vi "FPGA.vi"() -> ()   [LabVIEW 2017]
uses:
  <vilib>/Platform/TimedLoop/XDataNode/timing_clust.ctl
  <vilib>/Platform/TimedLoop/XDataNode/nitl_modes.ctl
  <vilib>/Platform/TimedLoop/XDataNode/wakeup.ctl
  <vilib>/rvi/Emulation/niFpgaGetClockAttributes.vi
  <vilib>/rvi/Emulation/niFpgaSctlEmulationGetInTimedLoop.vi
  <vilib>/rvi/Emulation/niFpgaEmulationReportErrorSimple.vi
  <vilib>/rvi/eio/common/nirviEmuTemplateMethod_errors.vi
  <vilib>/rvi/Emulation/niFpgaCriticalErrorInLSC.vi
  <vilib>/rvi/Emulation/niFpgaProcessEmulError.vi
  Control/GV FIFO timeout.vi
  Control/GV DO delay.vi
  Control/GV trigger delay.vi
  <vilib>/eio/EIONode/EIONode.xnode
  <vilib>/Platform/TimedLoop/XDataNode/XDataNode.xnode
  <vilib>/Platform/TimedLoop/XDataNode/XDNodeRunTimeDep.lvlib
  <vilib>/rvi/occurrence/nirviOccurrence.lvlib
  Detector/GV gated pixel clock change.vi
  Detector/GV line gate.vi
  Detector/GV pretrigger.vi
panel:
  in  "FIFO OUT debug":bool
  in  "PC1_voltage":i16
  in  "RS_voltage":i16
  in  "ON/OFF":bool
  in  "VT_NC":bool
  in  "VT_forward":bool
  in  "VT_back":bool
  in  "VT_start":bool
  in  "Sync_AODO_to_LineGate":u16
  in  "Start_acquisition":bool
  in  "Nmax_lines":u16=1
  in  "Pulse sequence":bool[](array[boolean])=[TRUE, FALSE, FALSE, FALSE, FALSE, FALSE, FALSE, FALSE, FALSE, FALSE, FALSE, FALSE, FALSE, FALSE, FALSE, FALSE, FALSE, FALSE, FALSE, FALSE]
  in  "Nchannels":u16=4
  in  "FIFO_timeout":u16=100
  in  "Trigger":bool
  in  "Sync_DO_to_AO":u16=296
  # "RESONANT\nSCANNER"
  # "POCKELS #1"
  # "VIBRATOME"
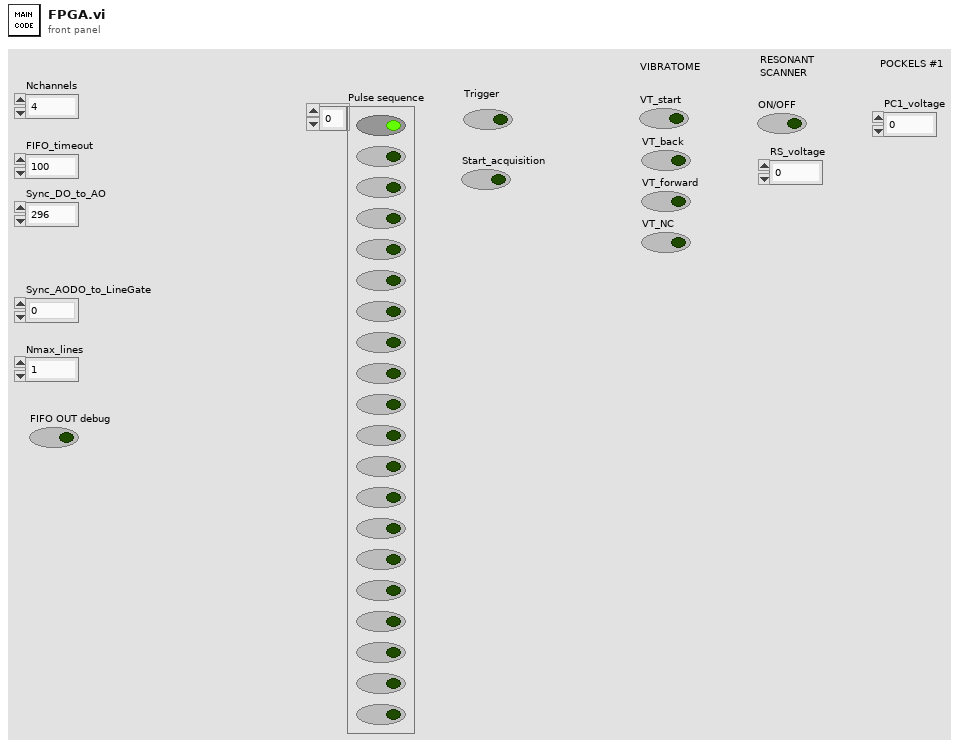
[diagram p1: front panel]
types:
  T1 = typedef "XDNodeRunTimeDep.lvlib/timing_clust.ctl" = cluster{"Expected End [f-1]":u64, "Actual End [f-1]":u64, "Finished Late? [f-1]":bool, "Expected End [i-1]":u64, "Actual End [i-1]":u64, "Finished Late? [i-1]":bool, "Expected Start [i]":u64, "Actual Start [i]":u64, "Expected Start [f]":u64, "Actual Start [f]":u64, "Source Name":string, "Structure Name":string, "Period":i64, "Deadline":i64, "Offset":i64, "Start":i64, "Priority":i32, "Timeout":i32, "Mode":T2, "Wakeup Reason":T3, "Error":errorcluster, "Source Type":string, "Secondary Source Type":string, "Global End Time":u64, "Global Start Time":u64, "Frame Duration":u64, "Iteration Duration":u64, "Assigned CPU":i32, "I/O Scan Engine Mode":u32}
  T2 = typedef "XDNodeRunTimeDep.lvlib/nitl_modes.ctl" = enum32{"No Change", "Process missed periods, maintain original phase", "Discard missed periods, maintain original phase", "Process missed periods, ignore original phase", "Discard missed periods, ignore original phase"}
  T3 = typedef "XDNodeRunTimeDep.lvlib/wakeup.ctl" = enum32{"Normal", "Aborted", "Asynchronous wakeup", "Timing source error", "Timed loop error", "Timeout"}
  T4 = cluster{"Pixel clock change":bool, "Line clock change":bool}
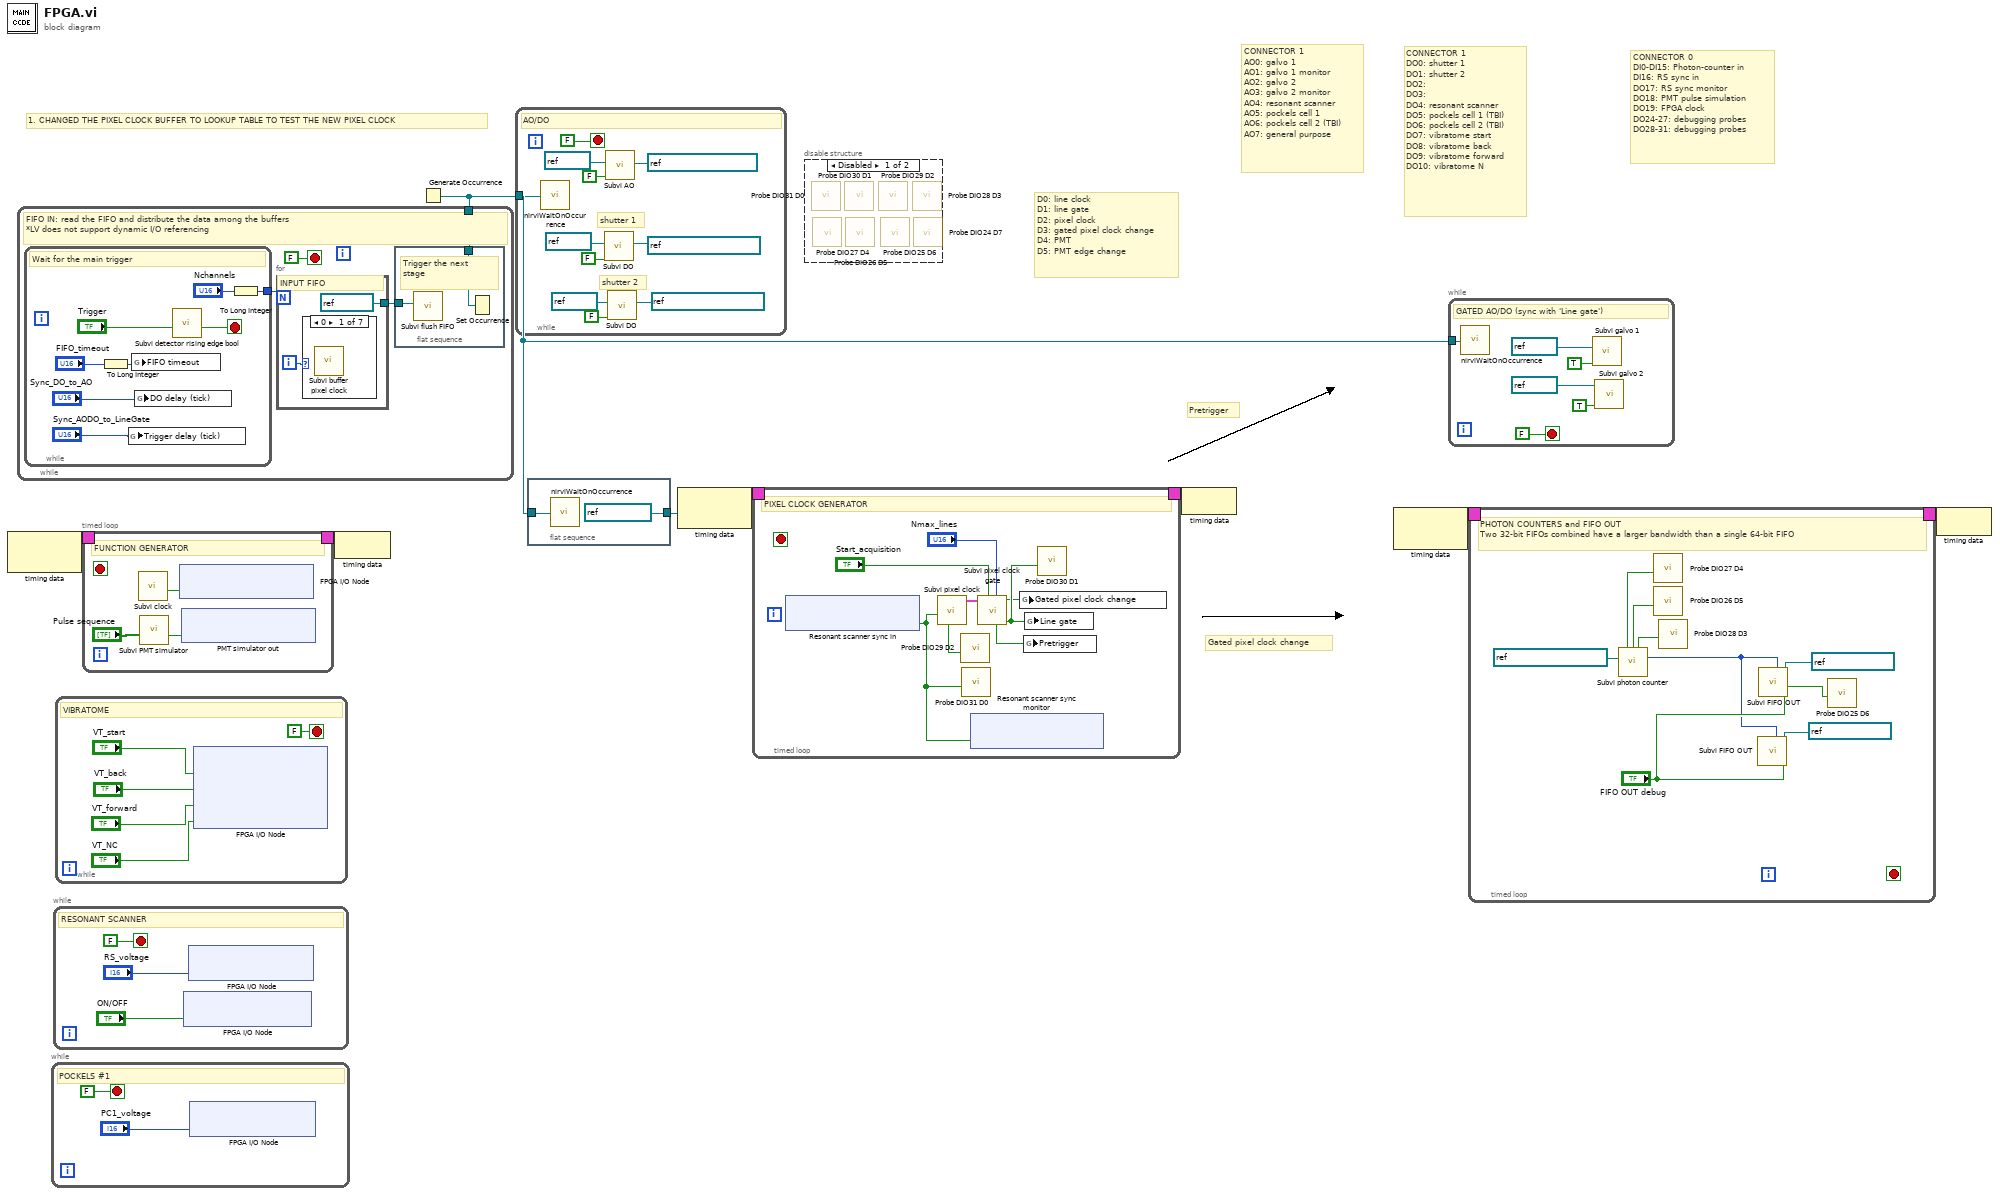
[diagram p0: block diagram]
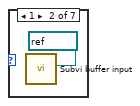
[diagram p3: hidden frame]
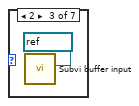
[diagram p4: hidden frame]
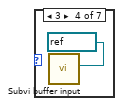
[diagram p5: hidden frame]
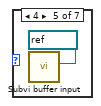
[diagram p6: hidden frame]
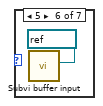
[diagram p7: hidden frame]
diagram:
  # "CONNECTOR 0\nDI0-DI15: Photon-counter in\nDI16: RS sync in \nDO17: RS sync monitor\nDO18: PMT pulse simulation\nDO19: FPGA clock\nDO24-27: debugging probes\nDO28-31: debugging probes"
  # "CONNECTOR 1\nDO0: shutter 1\nDO1: shutter 2\nDO2: \nDO3:\nDO4: resonant scanner\nDO5: pockels cell 1 (TBI)\nDO6: pockels cell 2 (TBI)\nDO7: vibratome start\nDO8: vibratome back\nDO9: vibratome forward\nDO10: vibratome N"
  # "CONNECTOR 1\nAO0: galvo 1\nAO1: galvo 1 monitor\nAO2: galvo 2\nAO3: galvo 2 monitor\nAO4: resonant scanner\nAO5: pockels cell 1\nAO6: pockels cell 2 (TBI)\nAO7: general purpose"
  # "D0: line clock\nD1: line gate\nD2: pixel clock\nD3: gated pixel clock change\nD4: PMT\nD5: PMT edge change"
  # "Gated pixel clock change"
  # "Pretrigger"
  # "1. CHANGED THE PIXEL CLOCK BUFFER TO LOOKUP TABLE TO TEST THE NEW PIXEL CLOCK"
  n1 = node-c288() -> (w3:T1)  [unwired: 1 in]
  n2 = while {
    stop <- FALSE stop-if-true
    # "POCKELS #1"
    n3 = xnode "FPGA I/O Node"("Connector1/AO5"="PC1_voltage") -> ()  [unwired: 1 in, 1 out]
  }
  n4 = while {
    stop <- FALSE stop-if-true
    # "RESONANT SCANNER"
    n5 = xnode "FPGA I/O Node"("Connector1/DIO4"="ON/OFF") -> ()  [unwired: 1 in, 1 out]
    n6 = xnode "FPGA I/O Node"("Connector1/AO4"="RS_voltage") -> ()  [unwired: 1 in, 1 out]
  }
  n7 = while {
    stop <- FALSE stop-if-true
    # "VIBRATOME"
    n8 = xnode "FPGA I/O Node"("Connector1/DIO7"="VT_start", "Connector1/DIO8"="VT_back", "Connector1/DIO9"="VT_forward", "Connector1/DIO10"="VT_NC") -> ()  [unwired: 4 in, 4 out]
  }
  n9 = timed-loop {
    timing: w3 -> [_]
    timing-out: [_] -> w2
    stop <- _ stop-if-true
    # "FUNCTION GENERATOR"
    n10 = call "Subvi clock.vi"() -> ("Output"=w21:bool)  [unwired: 11 in]
    n11 = call "Subvi PMT simulator.vi"("Pulse sequence"="Pulse sequence") -> ("output"=w19:bool)  [unwired: 10 in]
    n12 = xnode "FPGA I/O Node"("Connector0/DIO19"=w21) -> ()  [unwired: 1 in, 1 out]
    n13 = xnode ("PMT simulator out")("Connector0/DIO18"=w19) -> ()  [unwired: 1 in, 1 out]
  }
  n14 = node-c288(w2) -> ()
  n15 = Generate Occurrence() -> (w1:refnum<k4>)
  n16 = while {
    tunnel: w1 -> [w24]
    stop <- FALSE stop-if-true
    # "FIFO IN: read the FIFO and distribute the data among the buffers\n*LV does not support dynamic I/O referencing"
    n17 = while {
      tunnel: [w37] -> w26
      stop <- w44 stop-if-true
      # "Wait for the main trigger"
      n18 = To Long Integer(number="FIFO_timeout") -> (32bit integer=w38:i32)
      n19 = global write "GV trigger delay.vi" "Trigger delay (tick)"("Sync_AODO_to_LineGate") -> ()
      n20 = global write "GV FIFO timeout.vi" "FIFO timeout"(w38) -> ()
      n21 = global write "GV DO delay.vi" "DO delay (tick)"("Sync_DO_to_AO") -> ()
      n22 = call "Subvi detector rising edge bool.vi"("Input"="Trigger") -> ("Output"=w44:bool)  [unwired: 10 in]
      n23 = To Long Integer(number="Nchannels") -> (32bit integer=w37:i32)
    }
    n24 = for {
      N: w26 -> [_]
      tunnel: [refnum<k21> "FIFO IN" ("FIFO In")] -> w25
      i -> [w31]
      # "INPUT FIFO"
      n25 = case shown="0" w31 {
        frame 0 {
          n26 = call "Subvi buffer pixel clock.vi"() -> ()  [unwired: 12 in]
        }
        frame 1 {
          n27 = call "Subvi buffer input.vi"("Buffers"=refnum<k21> "AB0" ("FIFO In")) -> ()  [unwired: 11 in]
        }
        frame 2 {
          n28 = call "Subvi buffer input.vi"("Buffers"=refnum<k21> "AB1" ("FIFO In")) -> ()  [unwired: 11 in]
        }
        frame 3 {
          n29 = call "Subvi buffer input.vi"("Buffers"=refnum<k21> "AB2" ("FIFO In")) -> ()  [unwired: 11 in]
        }
        frame 4 {
          n30 = call "Subvi buffer input.vi"("Buffers"=refnum<k21> "DB0" ("FIFO In")) -> ()  [unwired: 11 in]
        }
        frame 5 {
          n31 = call "Subvi buffer input.vi"("Buffers"=refnum<k21> "DB1" ("FIFO In")) -> ()  [unwired: 11 in]
        }
        frame -1, Default {
        }
      }
    }
    n32 = flat-sequence {
      tunnel: w25 -> [w29]
      tunnel: w24 -> [w28]
      frame #0 {
        # "Trigger the next stage"
        n33 = call "Subvi flush FIFO.vi"("FIFO In"=w29) -> ()  [unwired: 10 in]
        n34 = Set Occurrence(w28) -> ()
      }
    }
  }
  n35 = while {
    tunnel: w1 -> [w54]
    stop <- FALSE stop-if-true
    # "shutter 2"
    # "shutter 1"
    # "AO/DO"
    n36 = call <vilib>:"nirviWaitOnOccurrence.vi"("occurrence"=w54) -> ()  [unwired: 4 in, 1 out]
    n37 = call "Subvi DO.vi"("DO"=refnum<k21> "Connector1/DIO0", "Ext trig enable"=FALSE, "FIFO In"=refnum<k21> "DB0") -> ()  [unwired: 9 in]
    n38 = call "Subvi AO.vi"("AO"=refnum<k21> "Connector1/AO7", "Ext trig enable"=FALSE, "FIFO In"=refnum<k21> "AB2") -> ()  [unwired: 9 in]
    n39 = call "Subvi DO.vi"("DO"=refnum<k21> "Connector1/DIO1", "Ext trig enable"=FALSE, "FIFO In"=refnum<k21> "DB1") -> ()  [unwired: 9 in]
  }
  n40 = flat-sequence {
    tunnel: [refnum<k21> "160MHz" ("Source Name")] -> w6
    tunnel: w1 -> [w56]
    frame #0 {
      n41 = call <vilib>:"nirviWaitOnOccurrence.vi"("occurrence"=w56) -> ()  [unwired: 4 in, 1 out]
    }
  }
  n42 = node-c288(w6) -> (w8:T1)
  n43 = timed-loop {
    timing: w8 -> [_]
    timing-out: [_] -> w7
    stop <- _ stop-if-true
    # "PIXEL CLOCK GENERATOR"
    n44 = xnode "Resonant scanner sync in"() -> ("Connector0/DIO16"=w60:bool)  [unwired: 1 in, 1 out]
    n45 = call "Subvi pixel clock.vi"("Line clock"=w60) -> ("Pixel clock change/line clock change/FIFO OUT gate"=w65:T4, "Pixel clock mon"=w59:bool)  [unwired: 9 in]
    n46 = call "Probe DIO29 D2.vi"("D2"=w59) -> ()  [unwired: 11 in]
    n47 = call "Probe DIO31 D0.vi"("D0"=w60) -> ()  [unwired: 11 in]
    n48 = xnode "Resonant scanner sync monitor"("Connector0/DIO17"=w60) -> ()  [unwired: 1 in, 1 out]
    n49 = call "Subvi pixel clock gate.vi"("Nmax lines"="Nmax_lines", "Start_acquisition"="Start_acquisition", "Pixel clock change/line clock change"=w65) -> ("Line gate"=w62:bool, "Gated pixel clock change"=w58:bool, "Pretrigger"=w63:bool)  [unwired: 6 in]
    n50 = global write "GV gated pixel clock change.vi" "Gated pixel clock change"(w58) -> ()
    n51 = global write "GV pretrigger.vi" "Pretrigger"(w63) -> ()
    n52 = global write "GV line gate.vi" "Line gate"(w62) -> ()
    n53 = call "Probe DIO30 D1.vi"("D1"=w62) -> ()  [unwired: 11 in]
  }
  n54 = disable-structure shown="Disabled" {
    frame Disabled {
      n55 = call "Probe DIO31 D0.vi"() -> ()  [unwired: 12 in]
      n56 = call "Probe DIO27 D4.vi"() -> ()  [unwired: 12 in]
      n57 = call "Probe DIO30 D1.vi"() -> ()  [unwired: 12 in]
      n58 = call "Probe DIO26 D5.vi"() -> ()  [unwired: 12 in]
      n59 = call "Probe DIO29 D2.vi"() -> ()  [unwired: 12 in]
      n60 = call "Probe DIO25 D6.vi"() -> ()  [unwired: 12 in]
      n61 = call "Probe DIO28 D3.vi"() -> ()  [unwired: 12 in]
      n62 = call "Probe DIO24 D7.vi"() -> ()  [unwired: 12 in]
    }
    frame Enabled {
    }
  }
  n63 = node-c288(w7) -> ()
  n64 = node-c288() -> (w5:T1)  [unwired: 1 in]
  n65 = while {
    tunnel: w1 -> [w72]
    stop <- FALSE stop-if-true
    # "GATED AO/DO (sync with 'Line gate')"
    n66 = call <vilib>:"nirviWaitOnOccurrence.vi"("occurrence"=w72) -> ()  [unwired: 4 in, 1 out]
    n67 = call "Subvi galvo 1.vi"("Ext trig enable"=TRUE, "FIFO In"=refnum<k21> "AB0") -> ()  [unwired: 10 in]
    n68 = call "Subvi galvo 2.vi"("Ext trig enable"=TRUE, "FIFO In"=refnum<k21> "AB1") -> ()  [unwired: 10 in]
  }
  n69 = timed-loop {
    timing: w5 -> [_]
    timing-out: [_] -> w4
    stop <- _ stop-if-true
    # "PHOTON COUNTERS and FIFO OUT\nTwo 32-bit FIFOs combined have a larger bandwidth than a single 64-bit FIFO"
    n70 = call "Subvi photon counter.vi"("DI channel"=refnum<k21> "Connector0/DIO0") -> ("PMT mon"=w78:bool, "PMT edge change mon"=w77:bool, "Gated pixel clock change mon"=w75:bool, "Count"=w74:u8)  [unwired: 11 in]
    n71 = call "Probe DIO27 D4.vi"("D4"=w78) -> ()  [unwired: 11 in]
    n72 = call "Probe DIO26 D5.vi"("D5"=w77) -> ()  [unwired: 11 in]
    n73 = call "Probe DIO28 D3.vi"("D3"=w75) -> ()  [unwired: 11 in]
    n74 = call "Subvi FIFO OUT.vi"("FIFO OUT debug"="FIFO OUT debug", "FIFO OUT"=refnum<k21> "FIFO OUT b", "number 1"=w74) -> ()  [unwired: 8 in, 1 out]
    n75 = call "Subvi FIFO OUT.vi"("FIFO OUT debug"="FIFO OUT debug", "FIFO OUT"=refnum<k21> "FIFO OUT a", "number 1"=w74) -> ("Save element mon"=w76:bool)  [unwired: 8 in]
    n76 = call "Probe DIO25 D6.vi"("D6"=w76) -> ()  [unwired: 11 in]
  }
  n77 = node-c288(w4) -> ()
